vi "asyncAcq_occurenceRef_timeStamp_viServer.vi"(0 "reference":refnum<class "OSA300.lvclass">, 5 "error in (no error)":errorcluster) -> (14 "reference out":refnum<class "OSA300.lvclass">, 15 "new spectrum":bool, 17 "new interferogram":bool, 19 "error out":errorcluster)   [LabVIEW 2010, in "OSA300.lvclass"]
doc: "SubVI to a <B>Thorlabs_OSA_64</B> object.\n\n[GOOP 1.0]"
uses:
  OSA300.lvclass
  OSA.lvclass
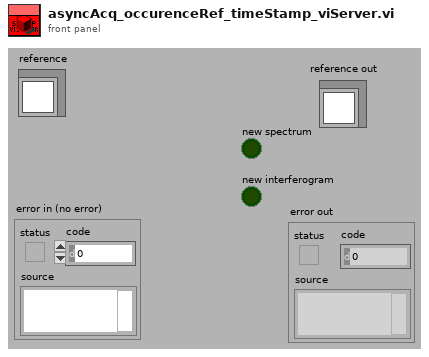
[diagram p1: front panel]
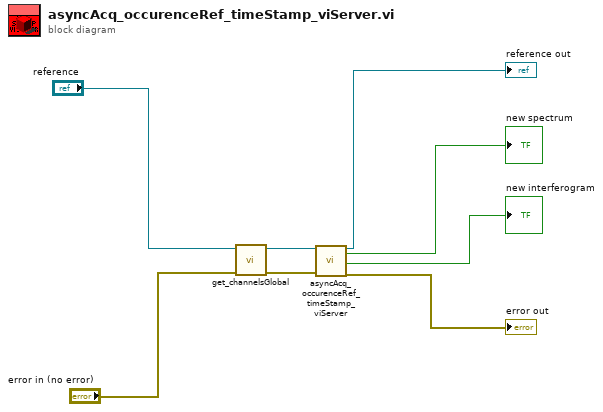
[diagram p0: block diagram]
diagram:
  n1 = call "get_channelsGlobal.vi"("error in (no error)"="error in (no error)", "OSA300 in"="reference") -> ("error out"=w1:errorcluster, "OSA300 out"=w2:refnum<class "OSA300.lvclass">)  [unwired: 8 in]
  n2 = call-parent "asyncAcq_occurenceRef_timeStamp_viServer.vi"("reference"=w2, "error in (no error)"=w1) -> ("reference out"=→"reference out":refnum<class "OSA300.lvclass">, "new spectrum"=→"new spectrum":bool, "new interferogram"=→"new interferogram":bool, "error out"=→"error out":errorcluster)  [unwired: 14 in]
